vi "Get RIO to APU Property Name.vi"(11 "rio name":string) -> (3 "property name":string)   [LabVIEW 2015, in "Engine Simulation Toolkit System Explorer.lvlib"]
uses:
  Engine Simulation Toolkit System Explorer.lvlib
  Shared/Properties.vi
  Shared/Engine Simulation Toolkit Shared.lvlib
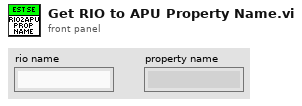
[diagram p1: front panel]
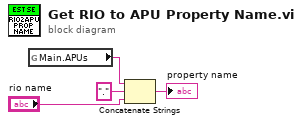
[diagram p0: block diagram]
diagram:
  n1 = global read "Properties.vi" "Main.APUs"() -> (w1:string)
  n2 = Concatenate Strings(w1, "." ("string"), "rio name") -> (→"property name":string)
